vi "VI Tree.vi"() -> ()   [LabVIEW 2016, in "Pfeiffer Vacuum.lvlib"]
doc: "Pfeiffer Vacuum Tree"
uses:
  Pfeiffer Vacuum.lvlib
panel:
  in  "choise":T1(ring)=enum."Handheld vacuum gauge"
  # "SEE DIAGRAM\nFOR VI TREE.\n\nTurbopumps\nOnTool DryPump\nDIGILINE\nHandheld Vacuum Gauge\nHLT 5xx\nMiniTest 300"
  # "Pfeiffer Vacuum GmbH . Berliner Strasse 43 . D-35614 Asslar\nTel.: +49 (0) 6441 802-0 . Fax: +49 (0) 6441 802-202\nwww.pfeiffer-vacuum.de"
  # "FPF"
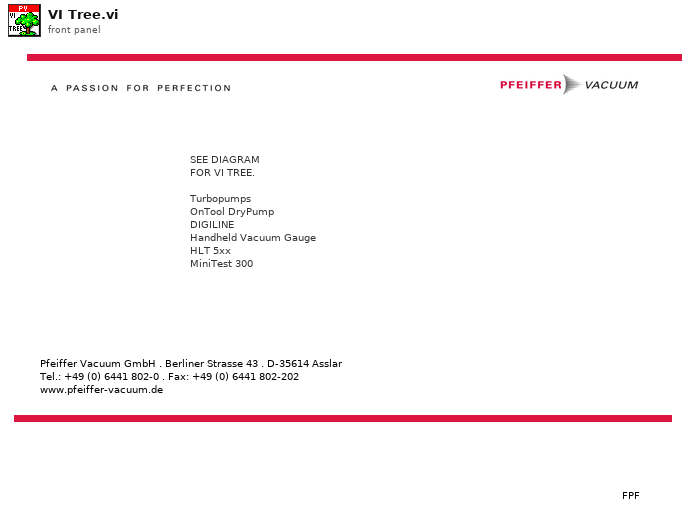
[diagram p1: front panel]
types:
  T1 = enum16{"Turbopump", "Digiline", "OnTool DryPump", "Handheld vacuum gauge", "MiniTest", "HLT 5xx"}
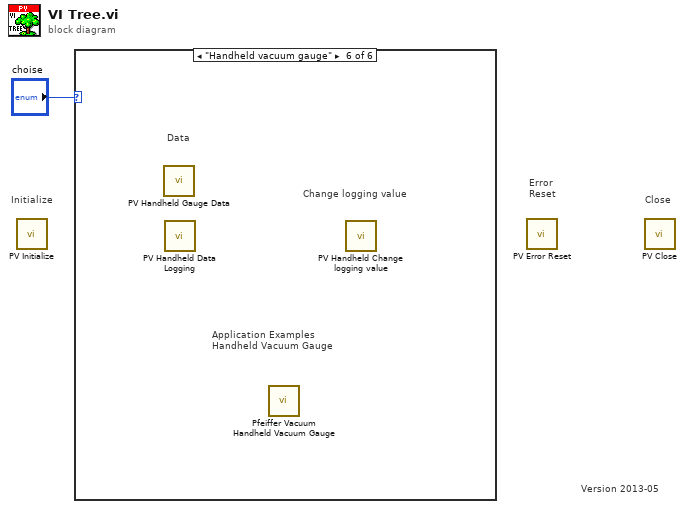
[diagram p0: block diagram]
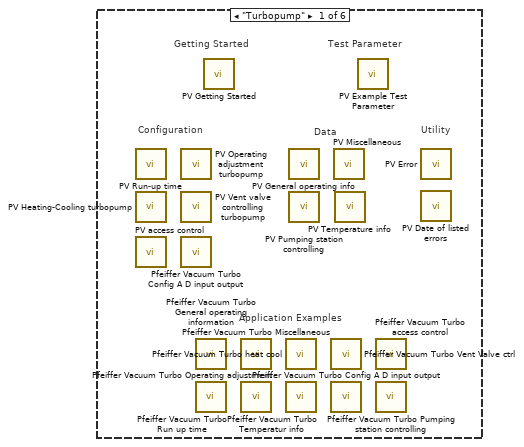
[diagram p2: hidden frame]
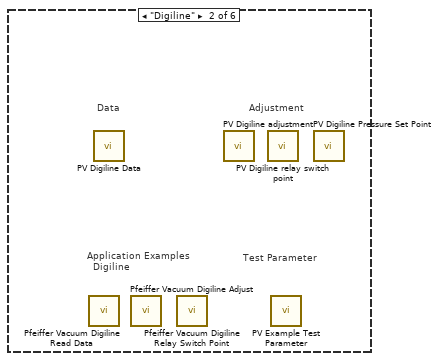
[diagram p3: hidden frame]
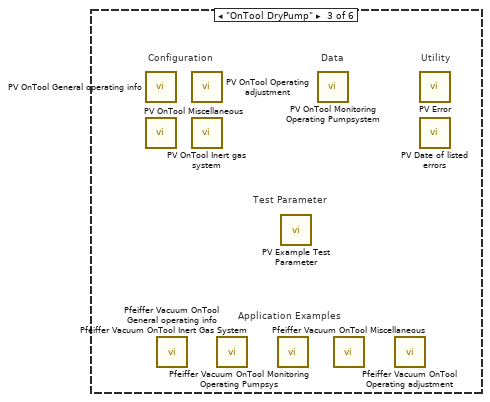
[diagram p4: hidden frame]
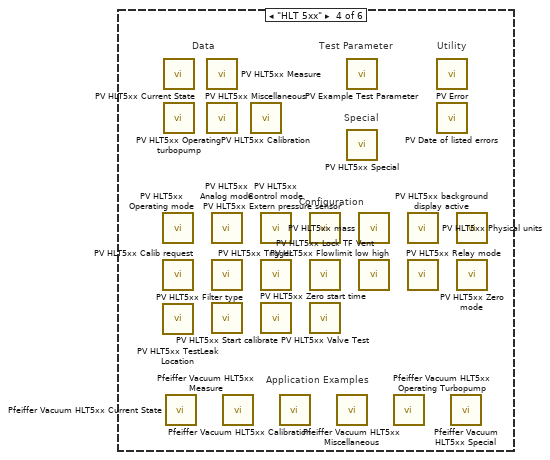
[diagram p5: hidden frame]
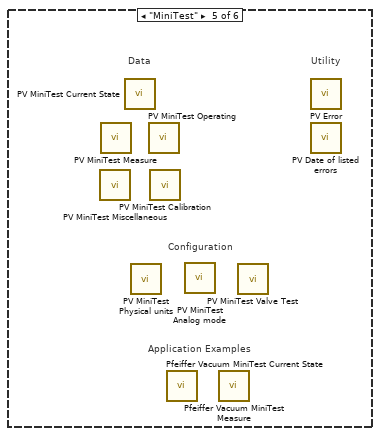
[diagram p6: hidden frame]
diagram:
  # "Error\nReset"
  # "Initialize"
  # "Version 2013-05"
  # "Close"
  n1 = call "PV Initialize.vi"() -> ()  [unwired: 10 in, 2 out]
  n2 = case shown="\"Handheld vacuum gauge\"" "choise" {
    frame "Turbopump" {
      # "Test Parameter"
      # "Getting Started"
      # "Data"
      # "Application Examples"
      # "Utility"
      # "Configuration"
      n3 = call "PV Run-up time.vi"() -> ()  [unwired: 9 in, 3 out]
      n4 = call "PV Heating-Cooling turbopump.vi"() -> ()  [unwired: 9 in, 3 out]
      n5 = call "PV access control.vi"() -> ()  [unwired: 8 in, 3 out]
      n6 = call "PV Operating adjustment turbopump.vi"() -> ()  [unwired: 9 in, 3 out]
      n7 = call "PV Vent valve controlling turbopump.vi"() -> ()  [unwired: 9 in, 3 out]
      n8 = call "Pfeiffer Vacuum Turbo Config A D input output.vi"() -> ()  [unwired: 10 in, 2 out]
      n9 = call "Pfeiffer Vacuum Turbo General operating information.vi"() -> ()  [unwired: 10 in, 2 out]
      n10 = call "Pfeiffer Vacuum Turbo Run up time.vi"() -> ()  [unwired: 10 in, 2 out]
      n11 = call "PV Getting Started.vi"() -> ()  [unwired: 13 in, 7 out]
      n12 = call "Pfeiffer Vacuum Turbo Miscellaneous.vi"() -> ()  [unwired: 10 in, 2 out]
      n13 = call "Pfeiffer Vacuum Turbo Operating adjustment.vi"() -> ()  [unwired: 10 in, 2 out]
      n14 = call "Pfeiffer Vacuum Turbo heat cool.vi"() -> ()  [unwired: 10 in, 2 out]
      n15 = call "Pfeiffer Vacuum Turbo Temperatur info.vi"() -> ()  [unwired: 10 in, 2 out]
      n16 = call "PV General operating info.vi"() -> ()  [unwired: 9 in, 3 out]
      n17 = call "PV Pumping station controlling.vi"() -> ()  [unwired: 9 in, 3 out]
      n18 = call "Pfeiffer Vacuum Turbo Vent Valve ctrl.vi"() -> ()  [unwired: 10 in, 2 out]
      n19 = call "Pfeiffer Vacuum Turbo Config A D input output.vi"() -> ()  [unwired: 10 in, 2 out]
      n20 = call "PV Miscellaneous.vi"() -> ()  [unwired: 9 in, 3 out]
      n21 = call "PV Temperature info.vi"() -> ()  [unwired: 13 in, 3 out]
      n22 = call "PV Example Test Parameter.vi"() -> ()  [unwired: 11 in, 1 out]
      n23 = call "Pfeiffer Vacuum Turbo access control.vi"() -> ()  [unwired: 10 in, 2 out]
      n24 = call "Pfeiffer Vacuum Turbo Pumping station controlling.vi"() -> ()  [unwired: 10 in, 2 out]
      n25 = call "PV Error.vi"() -> ()  [unwired: 8 in, 4 out]
      n26 = call "PV Date of listed errors.vi"() -> ()  [unwired: 13 in, 3 out]
    }
    frame "Digiline" {
      # "Test Parameter"
      # "Adjustment"
      # "Data"
      # "Application Examples\n  Digiline"
      n27 = call "Pfeiffer Vacuum Digiline Read Data.vi"() -> ()  [unwired: 10 in, 2 out]
      n28 = call "PV Digiline Data.vi"() -> ()  [unwired: 9 in, 3 out]
      n29 = call "Pfeiffer Vacuum Digiline Adjust.vi"() -> ()  [unwired: 10 in, 2 out]
      n30 = call "Pfeiffer Vacuum Digiline Relay Switch Point.vi"() -> ()  [unwired: 10 in, 2 out]
      n31 = call "PV Digiline adjustment.vi"() -> ()  [unwired: 9 in, 3 out]
      n32 = call "PV Digiline relay switch point.vi"() -> ()  [unwired: 9 in, 3 out]
      n33 = call "PV Example Test Parameter.vi"() -> ()  [unwired: 11 in, 1 out]
      n34 = call "PV Digiline Pressure Set Point.vi"() -> ()  [unwired: 10 in, 2 out]
    }
    frame "OnTool DryPump" {
      # "Test Parameter"
      # "Utility"
      # "Data"
      # "Configuration"
      # "Application Examples"
      n35 = call "PV OnTool General operating info.vi"() -> ()  [unwired: 13 in, 3 out]
      n36 = call "PV OnTool Miscellaneous.vi"() -> ()  [unwired: 9 in, 3 out]
      n37 = call "Pfeiffer Vacuum OnTool General operating info.vi"() -> ()  [unwired: 10 in, 2 out]
      n38 = call "PV OnTool Operating adjustment.vi"() -> ()  [unwired: 9 in, 3 out]
      n39 = call "PV OnTool Inert gas system.vi"() -> ()  [unwired: 9 in, 3 out]
      n40 = call "Pfeiffer Vacuum OnTool Inert Gas System.vi"() -> ()  [unwired: 10 in, 2 out]
      n41 = call "Pfeiffer Vacuum OnTool Monitoring Operating Pumpsys.vi"() -> ()  [unwired: 10 in, 2 out]
      n42 = call "PV Example Test Parameter.vi"() -> ()  [unwired: 11 in, 1 out]
      n43 = call "PV OnTool Monitoring Operating Pumpsystem.vi"() -> ()  [unwired: 9 in, 3 out]
      n44 = call "Pfeiffer Vacuum OnTool Miscellaneous.vi"() -> ()  [unwired: 10 in, 2 out]
      n45 = call "Pfeiffer Vacuum OnTool Operating adjustment.vi"() -> ()  [unwired: 10 in, 2 out]
      n46 = call "PV Error.vi"() -> ()  [unwired: 8 in, 4 out]
      n47 = call "PV Date of listed errors.vi"() -> ()  [unwired: 13 in, 3 out]
    }
    frame "HLT 5xx" {
      # "Data"
      # "Configuration"
      # "Special"
      # "Test Parameter"
      # "Application Examples"
      # "Utility"
      n48 = call "PV HLT5xx Operating mode.vi"() -> ()  [unwired: 8 in, 4 out]
      n49 = call "PV HLT5xx Calib request.vi"() -> ()  [unwired: 8 in, 4 out]
      n50 = call "PV HLT5xx TestLeak Location.vi"() -> ()  [unwired: 8 in, 4 out]
      n51 = call "PV HLT5xx Current State.vi"() -> ()  [unwired: 8 in, 4 out]
      n52 = call "PV HLT5xx Operating turbopump.vi"() -> ()  [unwired: 9 in, 3 out]
      n53 = call "Pfeiffer Vacuum HLT5xx Current State.vi"() -> ()  [unwired: 10 in, 2 out]
      n54 = call "PV HLT5xx Measure.vi"() -> ()  [unwired: 9 in, 3 out]
      n55 = call "PV HLT5xx Miscellaneous.vi"() -> ()  [unwired: 9 in, 3 out]
      n56 = call "PV HLT5xx Analog mode.vi"() -> ()  [unwired: 7 in, 5 out]
      n57 = call "PV HLT5xx Filter type.vi"() -> ()  [unwired: 8 in, 4 out]
      n58 = call "PV HLT5xx Start calibrate.vi"() -> ()  [unwired: 9 in, 3 out]
      n59 = call "Pfeiffer Vacuum HLT5xx Measure.vi"() -> ()  [unwired: 10 in, 2 out]
      n60 = call "PV HLT5xx Calibration.vi"() -> ()  [unwired: 12 in, 4 out]
      n61 = call "PV HLT5xx Control mode.vi"() -> ()  [unwired: 8 in, 4 out]
      n62 = call "PV HLT5xx Trigger.vi"() -> ()  [unwired: 9 in, 3 out]
      n63 = call "PV HLT5xx Zero start time.vi"() -> ()  [unwired: 8 in, 4 out]
      n64 = call "Pfeiffer Vacuum HLT5xx Calibration.vi"() -> ()  [unwired: 13 in, 3 out]
      n65 = call "PV HLT5xx Extern pressure sensor.vi"() -> ()  [unwired: 8 in, 4 out]
      n66 = call "PV HLT5xx Lock TF Vent.vi"() -> ()  [unwired: 8 in, 4 out]
      n67 = call "PV HLT5xx Valve Test.vi"() -> ()  [unwired: 7 in, 5 out]
      n68 = call "Pfeiffer Vacuum HLT5xx Miscellaneous.vi"() -> ()  [unwired: 10 in, 2 out]
      n69 = call "PV Example Test Parameter.vi"() -> ()  [unwired: 11 in, 1 out]
      n70 = call "PV HLT5xx Special.vi"() -> ()  [unwired: 9 in, 3 out]
      n71 = call "PV HLT5xx mass.vi"() -> ()  [unwired: 8 in, 4 out]
      n72 = call "PV HLT5xx Flowlimit low high.vi"() -> ()  [unwired: 13 in, 3 out]
      n73 = call "Pfeiffer Vacuum HLT5xx Operating Turbopump.vi"() -> ()  [unwired: 10 in, 2 out]
      n74 = call "PV HLT5xx Physical units.vi"() -> ()  [unwired: 7 in, 5 out]
      n75 = call "PV HLT5xx Relay mode.vi"() -> ()  [unwired: 7 in, 5 out]
      n76 = call "PV Error.vi"() -> ()  [unwired: 8 in, 4 out]
      n77 = call "PV Date of listed errors.vi"() -> ()  [unwired: 13 in, 3 out]
      n78 = call "Pfeiffer Vacuum HLT5xx Special.vi"() -> ()  [unwired: 10 in, 2 out]
      n79 = call "PV HLT5xx background display active.vi"() -> ()  [unwired: 8 in, 4 out]
      n80 = call "PV HLT5xx Zero mode.vi"() -> ()  [unwired: 8 in, 4 out]
    }
    frame "MiniTest" {
      # "Application Examples"
      # "Configuration"
      # "Data"
      # "Utility"
      n81 = call "PV MiniTest Miscellaneous.vi"() -> ()  [unwired: 9 in, 3 out]
      n82 = call "PV MiniTest Measure.vi"() -> ()  [unwired: 9 in, 3 out]
      n83 = call "PV MiniTest Current State.vi"() -> ()  [unwired: 8 in, 4 out]
      n84 = call "PV MiniTest Physical units.vi"() -> ()  [unwired: 7 in, 5 out]
      n85 = call "PV MiniTest Operating.vi"() -> ()  [unwired: 9 in, 3 out]
      n86 = call "PV MiniTest Calibration.vi"() -> ()  [unwired: 13 in, 3 out]
      n87 = call "Pfeiffer Vacuum MiniTest Current State.vi"() -> ()  [unwired: 9 in, 3 out]
      n88 = call "PV MiniTest Analog mode.vi"() -> ()  [unwired: 7 in, 5 out]
      n89 = call "Pfeiffer Vacuum MiniTest Measure.vi"() -> ()  [unwired: 10 in, 2 out]
      n90 = call "PV MiniTest Valve Test.vi"() -> ()  [unwired: 9 in, 3 out]
      n91 = call "PV Error.vi"() -> ()  [unwired: 8 in, 4 out]
      n92 = call "PV Date of listed errors.vi"() -> ()  [unwired: 13 in, 3 out]
    }
    frame "Handheld vacuum gauge" {
      # "Application Examples\nHandheld Vacuum Gauge"
      # "Data"
      # "Change logging value"
      n93 = call "PV Handheld Gauge Data.vi"() -> ()  [unwired: 9 in, 3 out]
      n94 = call "PV Handheld Data Logging.vi"() -> ()  [unwired: 9 in, 3 out]
      n95 = call "Pfeiffer Vacuum Handheld Vacuum Gauge.vi"() -> ()  [unwired: 10 in, 2 out]
      n96 = call "PV Handheld Change logging value.vi"() -> ()  [unwired: 8 in, 4 out]
    }
  }
  n97 = call "PV Error Reset.vi"() -> ()  [unwired: 10 in, 2 out]
  n98 = call "PV Close.vi"() -> ()  [unwired: 15 in, 1 out]
